vi "圈圈叉叉.vi"() -> ()   [LabVIEW 2014]
panel:
  out "O 方贏":bool
  out "X 方贏":bool
  in  "Toggle turn":bool
  out "下個順序":string
  in  "操作介面":bool[][](array[boolean])=[[FALSE, FALSE, FALSE], [FALSE, FALSE, FALSE], [FALSE, FALSE, FALSE]]
  in  "start/new game":bool
  out "戰況面板":string[][](array[string])
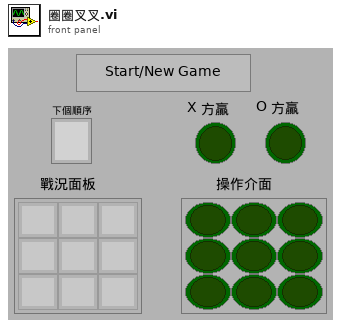
[diagram p1: front panel]
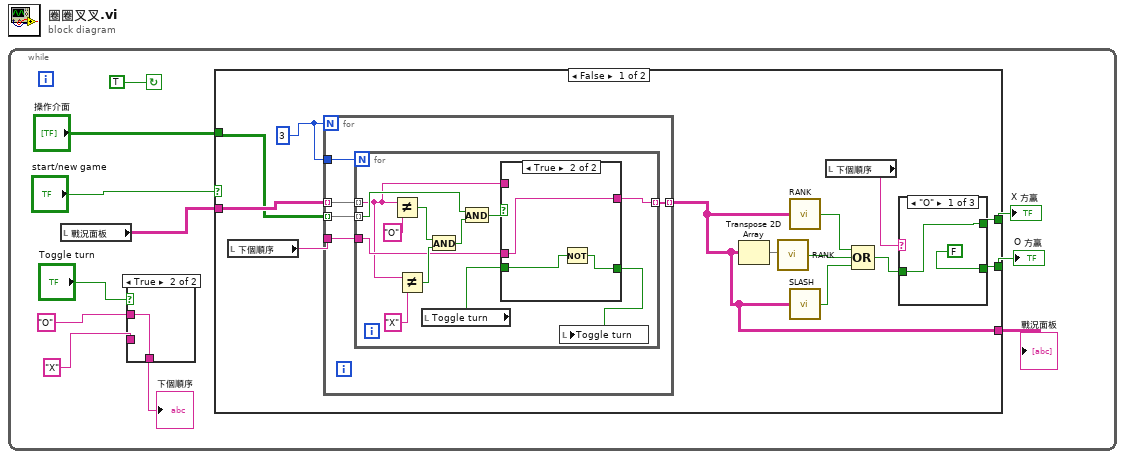
[diagram p0: block diagram]
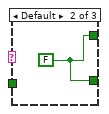
[diagram p3: hidden frame]
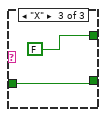
[diagram p4: hidden frame]
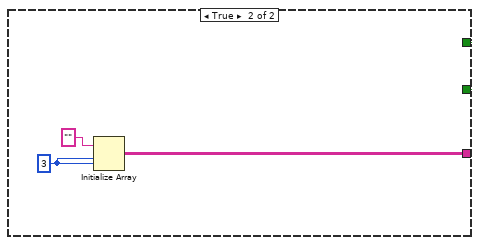
[diagram p6: hidden frame]
diagram:
  n1 = while {
    stop <- TRUE continue-if-true
    n2 = local read "戰況面板"() -> (w1:string[][])
    n3 = case shown="True" "Toggle turn" {
      tunnel: "O" -> [_ w13]
      tunnel: "X" -> [w12 _]
      tunnel: [w12 w13] -> w8
      frame False {
      }
      frame True {
      }
    }
    "下個順序" <- w8
    n4 = case shown="False" "start/new game" {
      tunnel: [w15 w58] -> w4
      tunnel: w1 -> [w24 _]
      tunnel: [w17 w54] -> w5
      tunnel: "操作介面" -> [w22 _]
      tunnel: [w16 w54] -> w3
      frame False {
        w26 = 3
        n5 = local read "下個順序"() -> (w25:string)
        n6 = for {
          N: w26 -> [_]
          tunnel: w26 -> [w36]
          tunnel: w22 -> [w35] mode=indexing
          tunnel: w25 -> [w33]
          tunnel: w24 -> [w34] mode=indexing
          tunnel: [w32] -> w15 mode=indexing
          n7 = for {
            N: w36 -> [_]
            tunnel: w35 -> [w43] mode=indexing
            tunnel: w33 -> [w42]
            tunnel: w34 -> [w40] mode=indexing
            tunnel: [w41] -> w32 mode=indexing
            n8 = Not Equal?(x=w40, y="O") -> (x != y?=w46:bool)
            n9 = Not Equal?(x=w40, y="X") -> (x != y?=w45:bool)
            n10 = local read "Toggle turn"() -> (w39:bool)
            n11 = And(x=w46, y=w45) -> (x .and. y?=w44:bool)
            n12 = And(x=w43, y=w44) -> (x .and. y?=w38:bool)
            n13 = case shown="True" w38 {
              tunnel: w42 -> [_ w51]
              tunnel: [w49 w51] -> w41
              tunnel: w40 -> [w49 _]
              tunnel: w39 -> [w50 w52]
              tunnel: [w50 w53] -> w37
              frame False {
              }
              frame True {
                n14 = Not(x=w52) -> (.not. x?=w53:bool)
              }
            }
            n15 = local write "Toggle turn"(w37) -> ()
          }
        }
        n16 = Transpose 2D Array(2D array=w15) -> (transposed array=w23:string[][])
        n17 = call "RANK.vi"("3*3陣列"=w23) -> ("O或X贏"=w19:bool)
        n18 = call "RANK.vi"("3*3陣列"=w15) -> ("O或X贏"=w20:bool)
        n19 = call "SLASH.vi"("3*3陣列"=w15) -> ("O或X贏"=w14:bool)
        n20 = local read "下個順序"() -> (w21:string)
        n21 = Compound Arithmetic op=OR(w20, w19, w14) -> (w18:bool)
        n22 = case shown="\"O\"" w21 {
          tunnel: [FALSE w29 w30] -> w16
          tunnel: [w27 w29 FALSE] -> w17
          tunnel: w18 -> [w27 _ w30]
          frame "O" {
          }
          frame Default {
            w29 = FALSE
          }
          frame "X" {
          }
        }
      }
      frame True {
        w56 = 3
        w54 = FALSE
        w60 = 3
        n23 = Initialize Array(FALSE, w56, w56) -> (w55:bool[][])
        n24 = Initialize Array("", w60, w60) -> (w58:string[][])
        n25 = local write "操作介面"(w55) -> ()
      }
    }
    "戰況面板" <- w4
    "X 方贏" <- w5
    "O 方贏" <- w3
  }
